vi "Global Property Names.vi"() -> ()   [LabVIEW 2011, in "Interpolate 1D Array Custom Device.lvlib"]
uses:
  Interpolate 1D Array Custom Device.lvlib
panel:
  in  "Spreadsheet Info":string="Spreadsheet Info"
  in  "Interpolate Options":string="Interpolate Options"
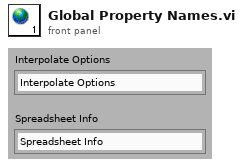
[diagram p1: front panel]
diagram:
